vi "Serialize.vi"(7 "DestinationFolder":path, 8 "error in":errorcluster, 9 "OwningElement in":refnum<k20>, 10 "Document in":refnum<k20>, 11 "SequenceRun in":refnum<class "SequenceRun.lvclass">) -> (0 "error out":errorcluster, 1 "OwningElement out":refnum<k20>, 2 "Document out":refnum<k20>, 3 "SequenceRun out":refnum<class "SequenceRun.lvclass">)   [LabVIEW 2021, in "ProligentXMLGenerator.lvlib" / "SequenceRun.lvclass"]
uses:
  SequenceRun.lvclass
  SequenceRun.lvclass/SequenceRun.ctl
  <vilib>/xml/NI_XML.lvlib
  Base/DOMSupport/DOMSupport.lvlib
  StepRun/StepRun/StepRun.lvclass
  Model/Characteristic/Characteristic.lvclass
  Model/Document/Document.lvclass
  Failure/FailureReference/FailureReference.lvclass
  Model/CustomData/CustomData.lvclass
  <vilib>/xml/Close Reference(Node).vi
  Base/DateTime/DateTime.lvclass
  C:/Projects/proligent-xml-generator-labview/src/ProligentXMLGenerator/Base/Attribute/Attribute.lvclass
  C:/Projects/proligent-xml-generator-labview/src/ProligentXMLGenerator/Base/DateTime/DateTime.lvclass
  Base/ExecutionStatus/ExecutionStatus.lvclass
  C:/Projects/proligent-xml-generator-labview/src/ProligentXMLGenerator/Base/ExecutionStatus/ExecutionStatus.lvclass
  Base/Guid/Guid.lvclass
  C:/Projects/proligent-xml-generator-labview/src/ProligentXMLGenerator/Base/NonEmptyString/NonEmptyString.lvclass
  C:/Projects/proligent-xml-generator-labview/src/ProligentXMLGenerator/Base/String/String.lvclass
  C:/Projects/proligent-xml-generator-labview/src/ProligentXMLGenerator/Base/Guid/Guid.lvclass
  Base/SequenceFullName/SequenceFullName.lvclass
  C:/Projects/proligent-xml-generator-labview/src/ProligentXMLGenerator/Base/SequenceFullName/SequenceFullName.lvclass
  Base/NonEmptyString_64/NonEmptyString_64.lvclass
  C:/Projects/proligent-xml-generator-labview/src/ProligentXMLGenerator/Base/NonEmptyString_64/NonEmptyString_64.lvclass
  Base/FullName/FullName.lvclass
  C:/Projects/proligent-xml-generator-labview/src/ProligentXMLGenerator/Base/FullName/FullName.lvclass
  Base/NonEmptyString_255/NonEmptyString_255.lvclass
  C:/Projects/proligent-xml-generator-labview/src/ProligentXMLGenerator/Base/NonEmptyString_255/NonEmptyString_255.lvclass
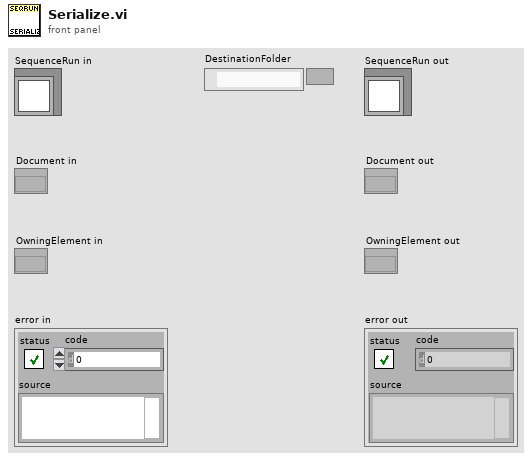
[diagram p1: front panel]
types:
  T1 = typedef "ProligentXMLGenerator.lvlib/SequenceRun.lvclass/Data.ctl" = cluster{"Name":string, "StepRuns":refnum<class "StepRun.lvclass">[], "Characteristics":refnum<class "Characteristic.lvclass">[], "Documents":refnum<class "Document.lvclass">[], "FailureReferences":refnum<class "FailureReference.lvclass">[], "CustomData":refnum<class "CustomData.lvclass">, "StartDate":refnum<class "DateTime.lvclass">, "EndDate":refnum<class "DateTime.lvclass">, "SequenceExecutionStatus":refnum<class "ExecutionStatus.lvclass">, "SequenceRunId":refnum<class "Guid.lvclass">, "SequenceFullName":refnum<class "SequenceFullName.lvclass">, "SequenceVersion":refnum<class "NonEmptyString_64.lvclass">, "StationFullName":refnum<class "FullName.lvclass">, "User":refnum<class "NonEmptyString_255.lvclass">, "TimeZoneInfoId":string}
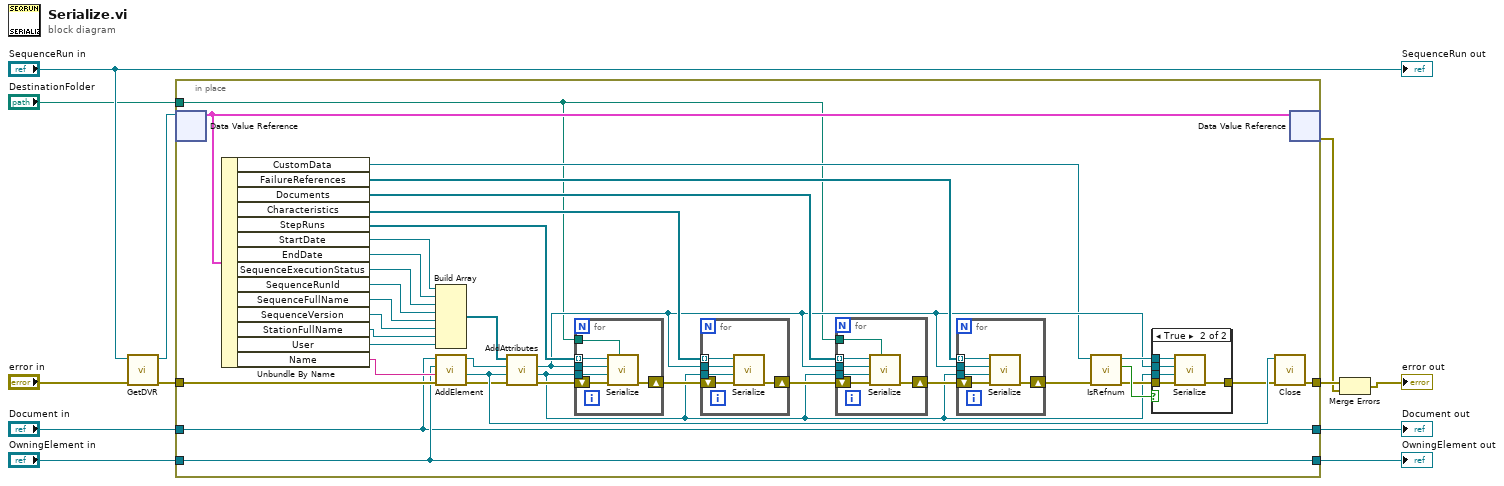
[diagram p0: block diagram]
diagram:
  n1 = call "GetDVR.vi"("error in"="error in", "SequenceRun"="SequenceRun in") -> ("error out"=w4:errorcluster, "DVRReference"=w3:refnum<data-value>)  [unwired: 8 in]
  n2 = in-place "In Place Element Structure" {
    in-place-border: [w47] -> w5
    in-place-border: "Document in" -> [w42]
    in-place-border: w4 -> [w46]
    in-place-border: "OwningElement in" -> [w44]
    in-place-border: [w44] -> w7
    in-place-border: [w42] -> w6
    in-place-border: "DestinationFolder" -> [w13]
    n3 = in-place-dvr #1(w3) -> (w43:T1)  [unwired: 1 out]
    n4 = Unbundle By Name(w43) -> ("CustomData"=w14:refnum<class "CustomData.lvclass">, "FailureReferences"=w25:refnum<class "FailureReference.lvclass">[], "Documents"=w26:refnum<class "Document.lvclass">[], "Characteristics"=w29:refnum<class "Characteristic.lvclass">[], "StepRuns"=w41:refnum<class "StepRun.lvclass">[], "StartDate"=w40:refnum<class "DateTime.lvclass">, "EndDate"=w39:refnum<class "DateTime.lvclass">, "SequenceExecutionStatus"=w38:refnum<class "ExecutionStatus.lvclass">, "SequenceRunId"=w24:refnum<class "Guid.lvclass">, "SequenceFullName"=w37:refnum<class "SequenceFullName.lvclass">, "SequenceVersion"=w22:refnum<class "NonEmptyString_64.lvclass">, "StationFullName"=w36:refnum<class "FullName.lvclass">, "User"=w23:refnum<class "NonEmptyString_255.lvclass">, "Name"=w45:string)
    n5 = Build Array(w40, w39, w38, w24, w37, w22, w36, w23) -> (w31:refnum<class "Attribute.lvclass">[])
    n6 = call "AddElement.vi"("error in"=w46, "Name"=w45, "OwningElement in"=w44, "Document in"=w42) -> ("error out"=w33:errorcluster, "NewElement"=w34:refnum<k20>, "Document out"=w35:refnum<k20>)  [unwired: 4 in, 1 out]
    n7 = call "AddAttributes.vi"("error in"=w33, "OwningElement in"=w34, "Document in"=w35, "Attributes"=w31) -> ("error out"=w32:errorcluster, "OwningElement out"=w16:refnum<k20>, "Document out"=w15:refnum<k20>)  [unwired: 5 in]
    n8 = for {
      tunnel: w41 -> [w75] mode=indexing
      tunnel: w16 -> [w73]
      tunnel: w15 -> [w74]
      shift-right: [w71] -> w30
      shift-left: w32 -> [w72]
      tunnel: w13 -> [w70]
      n9 = call "Serialize.vi"("DestinationFolder"=w70, "error in"=w72, "OwningElement in"=w73, "Document in"=w74, "StepRun in"=w75) -> ("error out"=w71:errorcluster)  [unwired: 3 in, 3 out]
    }
    n10 = for {
      tunnel: w29 -> [w69] mode=indexing
      tunnel: w16 -> [w67]
      tunnel: w15 -> [w68]
      shift-right: [w65] -> w28
      shift-left: w30 -> [w66]
      n11 = call "Serialize.vi"("error in"=w66, "OwningElement in"=w67, "Document in"=w68, "DocumentType in"=w69) -> ("error out"=w65:errorcluster)  [unwired: 4 in, 3 out]
    }
    n12 = for {
      tunnel: w26 -> [w64] mode=indexing
      tunnel: w16 -> [w62]
      tunnel: w15 -> [w63]
      shift-right: [w60] -> w27
      shift-left: w28 -> [w61]
      tunnel: w13 -> [w59]
      n13 = call "Serialize.vi"("DestinationFolder"=w59, "error in"=w61, "OwningElement in"=w62, "Document in"=w63, "DocumentType in"=w64) -> ("error out"=w60:errorcluster)  [unwired: 3 in, 3 out]
    }
    n14 = for {
      tunnel: w25 -> [w58] mode=indexing
      tunnel: w16 -> [w56]
      tunnel: w15 -> [w57]
      shift-right: [w54] -> w18
      shift-left: w27 -> [w55]
      n15 = call "Serialize.vi"("error in"=w55, "OwningElement in"=w56, "Document in"=w57, "FailureReference in"=w58) -> ("error out"=w54:errorcluster)  [unwired: 4 in, 3 out]
    }
    n16 = call "IsRefnum.vi"("error in"=w18, "CustomDataType in"=w14) -> ("error out"=w19:errorcluster, "IsRefnum"=w21:bool, "CustomDataType out"=w20:refnum<class "CustomData.lvclass">)  [unwired: 7 in]
    n17 = case shown="True" w21 {
      tunnel: w15 -> [_ w50]
      tunnel: w19 -> [w48 w53]
      tunnel: [w48 w52] -> w17
      tunnel: w20 -> [_ w51]
      tunnel: w16 -> [_ w49]
      frame False {
      }
      frame True {
        n18 = call "Serialize.vi"("error in"=w53, "OwningElement in"=w49, "Document in"=w50, "CustomDataType in"=w51) -> ("error out"=w52:errorcluster)  [unwired: 4 in, 3 out]
      }
    }
    n19 = call-poly <vilib>:"Close.vi"("error in (no error)"=w17, "node"=w34) -> ("error out"=w47:errorcluster)  [unwired: 7 in]
    n20 = in-place-dvr #1(w43) -> (w2:errorcluster)  [unwired: 1 out]
  }
  "Document out" <- w6
  "OwningElement out" <- w7
  n21 = Merge Errors(w5, w2) -> (→"error out":errorcluster)
  "SequenceRun out" <- "SequenceRun in"
